vi "Constructor.vi"(6 "ShadowColor":u32(colorbox)=9868950, 7 "Offset":i16, 8 "error in (no error)":errorcluster, 9 "Transparancy":i32, 10 "VI Refnum":refnum<vi>, 11 "Shadow in":refnum<class "Shadow.lvclass">) -> (0 "error out":errorcluster, 3 "Shadow out":refnum<class "Shadow.lvclass">)   [LabVIEW 2021, in "UIShadow.lvlib" / "Shadow.lvclass"]
uses:
  Shadow.lvclass
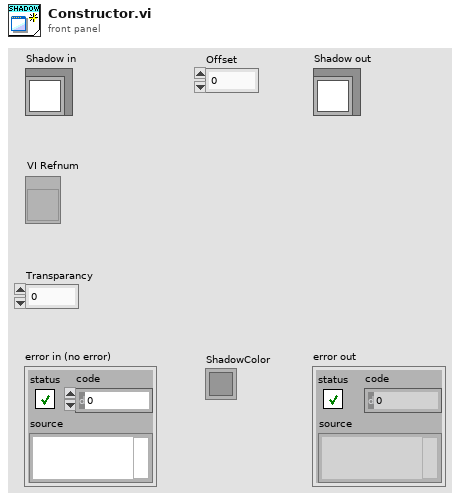
[diagram p1: front panel]
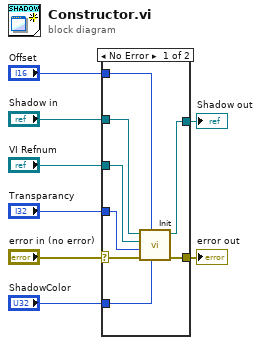
[diagram p0: block diagram]
diagram:
  n1 = case shown="No Error" "error in (no error)" {
    selector: "error in (no error)" -> [w16 w18]
    tunnel: [w15 w18] -> w7
    tunnel: [w13 w17] -> w5
    tunnel: "Shadow in" -> [w12 w17]
    tunnel: "VI Refnum" -> [w14 _]
    tunnel: "Transparancy" -> [w11 _]
    tunnel: "Offset" -> [w10 _]
    tunnel: "ShadowColor" -> [w9 _]
    frame No Error {
      n2 = call "Init.vi"("ShadowColor"=w9, "Offset"=w10, "error in (no error)"=w16, "Transparancy"=w11, "VI Refnum"=w14, "Shadow in"=w12) -> ("error out"=w15:errorcluster, "Shadow out"=w13:refnum<class "Shadow.lvclass">)  [unwired: 4 in]
    }
    frame Error {
    }
  }
  "error out" <- w7
  "Shadow out" <- w5
